vi "Set Step Evaluations.vi"(8 "error in (no error)":errorcluster, 9 "Evaluation Data":T1[](array[typedef]) {"Low Limit" format="%#_13g"; "SI Scaling" items=["femto"=-15, "pico"=-12, "nano"=-9, "micro"=-6, "milli"=-3, "percent"=-2, ""=0, "kilo"=3, "mega"=6, "giga"=9, "tera"=12]}, 10 "Step In":refnum<k7>, 11 "SPECAN_IQSLOT in":refnum<class "SPECAN_IQSLOT.lvclass">) -> (0 "error out":errorcluster, 2 "Step out":refnum<k7>, 3 "SPECAN_IQSLOT out":refnum<class "SPECAN_IQSLOT.lvclass">)   [LabVIEW 2018, in "SPECAN_IQSLOT.lvlib" / "SPECAN_IQSLOT.lvclass"]
uses:
  SPECAN_IQSLOT.lvclass
  C:/Sequence Automation/Plugins/Measurement Interface.lvlibp/Measurement Interface.lvclass
  Plugins/TestStand API Tools (TSAT).lvlibp/Evaluation Actions/Includes/Controls/TSAT Evaluation.ctl
  Plugins/TestStand API Tools (TSAT).lvlibp/Evaluation Actions/Includes/Controls/TSAT Eval SI Unit Scaling.ctl
  Plugins/TestStand API Tools (TSAT).lvlibp/Evaluation Actions/Includes/Controls/TSAT Evaluation Type.ctl
  Plugins/Measurement Interface.lvlibp/Private Methods/Engine Reference/Read Engine Reference.vi
  Plugins/TestStand API Tools (TSAT).lvlibp/Step Actions/TSAT Step Actions.lvlib
  Plugins/TestStand API Tools (TSAT).lvlibp/Evaluation Actions/TSAT Evaluation Actions.lvlib
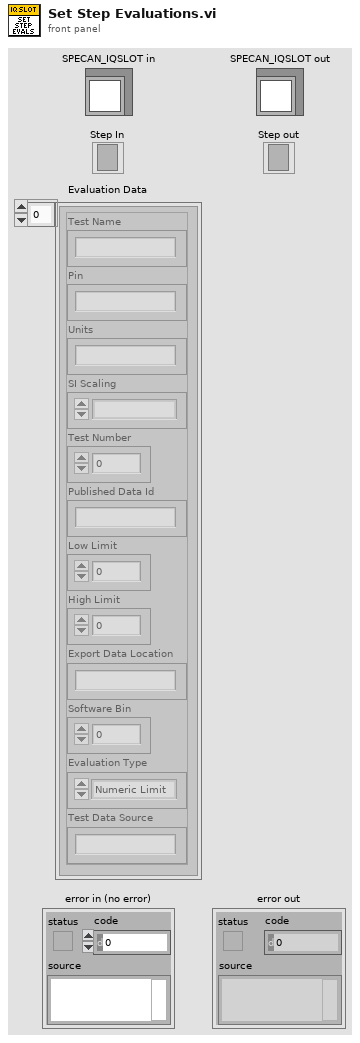
[diagram p1: front panel]
types:
  T1 = typedef "TestStand API Tools (TSAT).lvlibp/TSAT Evaluation Actions.lvlib/TSAT Evaluation.ctl" = cluster{"Test Name":string, "Pin":string, "Units":string, "SI Scaling":T2, "Test Number":i32, "Published Data Id":string, "Low Limit":dbl, "High Limit":dbl, "Export Data Location":string, "Software Bin":i64, "Evaluation Type":T3, "Test Data Source":string}
  T2 = typedef "TestStand API Tools (TSAT).lvlibp/TSAT Evaluation Actions.lvlib/TSAT Eval SI Unit Scaling.ctl" = i16
  T3 = typedef "TestStand API Tools (TSAT).lvlibp/TSAT Evaluation Actions.lvlib/TSAT Evaluation Type.ctl" = enum16{"Numeric Limit", "Pass/Fail", "None"}
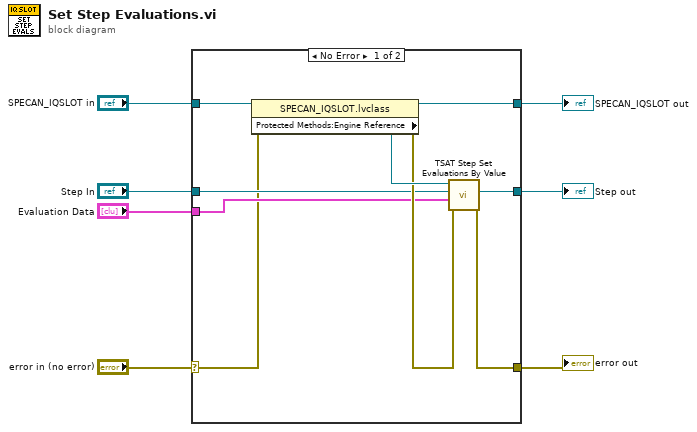
[diagram p0: block diagram]
diagram:
  n1 = case shown="No Error" "error in (no error)" {
    selector: "error in (no error)" -> [w8 w17]
    tunnel: "SPECAN_IQSLOT in" -> [w15 w19]
    tunnel: [w14 w19] -> w6
    tunnel: [w12 w17] -> w2
    tunnel: "Step In" -> [w11 w18]
    tunnel: "Evaluation Data" -> [w10 _]
    tunnel: [w9 w18] -> w1
    frame No Error {
      n2 = property class="SPECAN_IQSLOT.lvclass"(reference=w15, error in=w8) -> (reference out=w14:refnum<class "SPECAN_IQSLOT.lvclass">, error out=w13:errorcluster, "Protected Methods:Engine Reference"=w16:refnum<k7>)
      n3 = call "TSAT Step Set Evaluations By Value.vi"("Error In"=w13, "Evaluation Data"=w10, "Step In"=w11, "Engine In"=w16) -> ("Error Out"=w12:errorcluster, "Step Out"=w9:refnum<k7>)  [unwired: 5 in, 1 out]
    }
    frame Error {
    }
  }
  "error out" <- w2
  "SPECAN_IQSLOT out" <- w6
  "Step out" <- w1
